vi "Reset.vi"(7 "Reset to Default (False)":bool, 8 "error in (no error)":errorcluster, 11 "VISA resource name":refnum<visa-resource-name>) -> (0 "error out":errorcluster, 3 "VISA resource name out":refnum<visa-resource-name>)   [LabVIEW 2018, in "Lake Shore 372.lvlib"]
doc: "Resets the instrument and then sends a set of default setup commands to the instrument.\n\nNOTE: If you do not want the instrument reset to its default setup state you MUST set the Reset Defaults control to FALSE."
uses:
  Lake Shore 372.lvlib
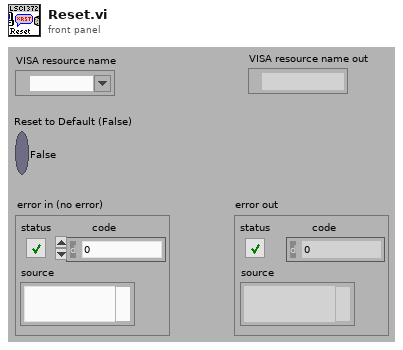
[diagram p1: front panel]
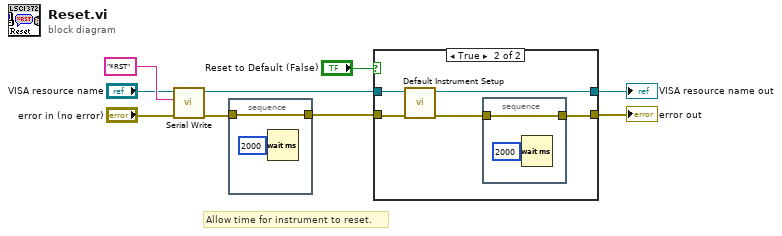
[diagram p0: block diagram]
diagram:
  # "Allow time for instrument to reset."
  n1 = call "Serial Write.vi"("error in (no error)"="error in (no error)", "Write Buffer (\"\")"="*RST" ("Reset Command"), "VISA resource name"="VISA resource name") -> ("error out"=w2:errorcluster, "VISA resource name out"=w1:refnum<visa-resource-name>)  [unwired: 6 in, 1 out]
  n2 = stacked-sequence {
    tunnel: w2 -> [w10]
    tunnel: [w10] -> w7
    frame #0 {
      n3 = Wait (ms)(milliseconds to wait=u32 2000) -> ()  [unwired: 1 out]
    }
  }
  n4 = case shown="True" "Reset to Default (False)" {
    tunnel: [w12 w14] -> w9
    tunnel: [w13 w16] -> w8
    tunnel: w7 -> [w12 w17]
    tunnel: w1 -> [w13 w18]
    frame False {
    }
    frame True {
      n5 = call "Default Instrument Setup.vi"("error in (no error)"=w17, "VISA resource name"=w18) -> ("error out"=w15:errorcluster, "VISA resource name out"=w16:refnum<visa-resource-name>)  [unwired: 8 in]
      n6 = stacked-sequence {
        tunnel: w15 -> [w19]
        tunnel: [w19] -> w14
        frame #0 {
          n7 = Wait (ms)(milliseconds to wait=u32 2000) -> ()  [unwired: 1 out]
        }
      }
    }
  }
  "error out" <- w9
  "VISA resource name out" <- w8
